vi "blfind_EChemEthDev.vi"(6 "error in (no error)":errorcluster, 9 "DLL Path":path) -> (0 "error out":errorcluster, 3 "device table":string[][](array[string]))   [LabVIEW 2022 SP3, in "EClib functions.lvlib"]
uses:
  EClib functions.lvlib
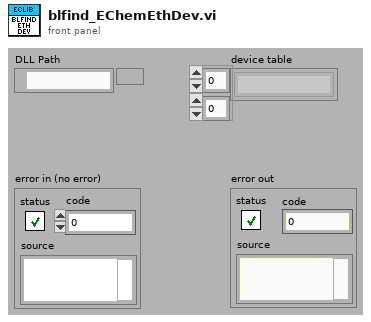
[diagram p1: front panel]
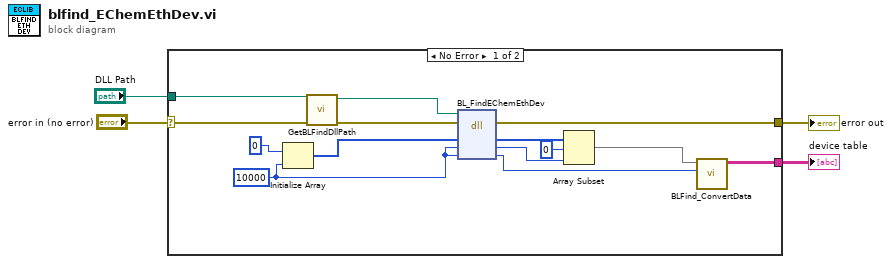
[diagram p0: block diagram]
diagram:
  n1 = case shown="No Error" "error in (no error)" {
    selector: "error in (no error)" -> [w9 w19]
    tunnel: [w6 w19] -> w3
    tunnel: [w10 _] -> w2
    tunnel: "DLL Path" -> [w5 _]
    frame No Error {
      w12 = 10000 ("dimension size")
      n2 = Initialize Array(u8 0, w12) -> (w14:u8[])
      n3 = call "GetBLFindDllPath.vi"("error in (no error)"=w9, "DLL Path"=w5) -> ("error out"=w7:errorcluster, "BlfindDLLPath"=w8:path)  [unwired: 8 in]
      n4 = dll-call lib="C:/EC-Lab Development Package/lib/blfind.dll" fn="BL_FindEChemEthDev"(path in=w8, error in=w7, "pLstdev"=w14, "psize"=w12, "pNbrDev"=w12) -> (error out=w6:errorcluster, "pLstdev"=w15:u16[], "psize"=w16:u32, "pNbrDev"=w17:u32)  [unwired: 2 in, 1 out]
      n5 = Array Subset(array=w15, index=0, length=w16) -> (w18:u16[])
      n6 = call "BLFind_ConvertData.vi"("pNbrDev"=w17, "pLstdev"=w18) -> ("device table"=w10:string[][])  [unwired: 9 in]
    }
    frame Error {
    }
  }
  "error out" <- w3
  "device table" <- w2
